vi "KE_Measure_Ir.vi"(0 "KE_In":refnum<visa-resource-name>, 1 "Samples":i32=1, 2 "Voltage":dbl, 3 "Compliance":dbl=0.1, 4 "SettleDelay":u32, 5 "error in (no error)":errorcluster) -> (6 "KE_Out":refnum<visa-resource-name>, 7 "Current(A)":dbl format="%0.2f", 8 "error out":errorcluster)   [LabVIEW 2012]
uses:
  <instrlib>/Keithley 24XX/Public/Data/Read (Multiple Points).vi
  <vilib>/Analysis/baseanly.llb/Mean (DBL).vi
  <instrlib>/Keithley 24XX/Keithley 24XX.lvlib
  <vilib>/Analysis/NI_AALBase.lvlib
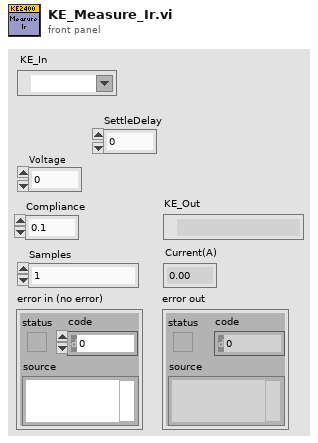
[diagram p1: front panel]
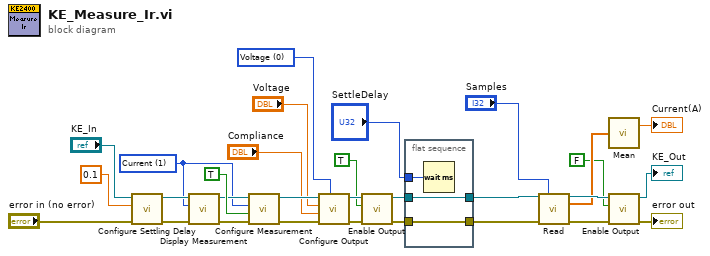
[diagram p0: block diagram]
diagram:
  w8 = u16 1 items=["Volts", "Current", "Resistance"] ("Function (0: Volts)")
  w23 = u16 0 items=["Voltage", "Current"] ("Source Mode  (0: Voltage)")
  n1 = call <instrlib>:"Configure Settling Delay.vi"("error in (no error)"="error in (no error)", "Manual Settling Delay (0 sec)"=0.1, "VISA resource name"="KE_In") -> ("error out"=w11:errorcluster, "VISA resource name out"=w13:refnum<visa-resource-name>)  [unwired: 7 in]
  n2 = call <instrlib>:"Display Measurement.vi"("error in (no error)"=w11, "Displayed Measurement (0: Voltage)"=w8, "VISA resource name"=w13) -> ("error out"=w7:errorcluster, "VISA resource name out"=w10:refnum<visa-resource-name>)  [unwired: 7 in]
  n3 = call <instrlib>:"Configure Measurement.vi"("error in (no error)"=w7, "Enable Auto Range (T:Enable)"=TRUE, "Function (0: Volts)"=w8, "VISA resource name"=w10) -> ("error out"=w27:errorcluster, "VISA resource name out"=w28:refnum<visa-resource-name>)  [unwired: 6 in]
  n4 = call <instrlib>:"Configure Output.vi"("Source Mode  (0: Voltage)"=w23, "error in (no error)"=w27, "Compliance  Level (0.1)"="Compliance", "Output Level (0)"="Voltage", "VISA resource name"=w28) -> ("error out"=w29:errorcluster, "VISA resource name out"=w30:refnum<visa-resource-name>)  [unwired: 5 in]
  n5 = call <instrlib>:"Enable Output.vi"("error in (no error)"=w29, "Enable Output (T: Enable)"=TRUE, "VISA resource name"=w30) -> ("error out"=w2:errorcluster, "VISA resource name out"=w3:refnum<visa-resource-name>)  [unwired: 7 in]
  n6 = flat-sequence {
    tunnel: "SettleDelay" -> [w33]
    tunnel: [w32] -> w4
    tunnel: w3 -> [w32]
    tunnel: w2 -> [w31]
    tunnel: [w31] -> w1
    frame #0 {
      n7 = Wait (ms)(milliseconds to wait=w33) -> ()  [unwired: 1 out]
    }
  }
  n8 = call-poly <instrlib>:"Read.vi"("VISA resource name"=w4, "Sample Count (1)"="Samples", "error in (no error)"=w1) -> ("VISA resource name out"=w20:refnum<visa-resource-name>, "Current"=w15:sgl[], "error out"=w19:errorcluster)  [unwired: 6 in, 4 out]
  n9 = call-poly <vilib>:"Mean.vi"("X"=w15) -> ("mean"=→"Current(A)":dbl)  [unwired: 1 out]
  n10 = call <instrlib>:"Enable Output.vi"("error in (no error)"=w19, "Enable Output (T: Enable)"=FALSE, "VISA resource name"=w20) -> ("error out"=→"error out":errorcluster, "VISA resource name out"=→"KE_Out":refnum<visa-resource-name>)  [unwired: 7 in]
